vi "cv_03-03.vi"() -> ()   [LabVIEW 2013]
panel:
  out "SR - 3":dbl
  out "SR - 2":dbl
  out "SR - 1":dbl
  out "Feedback Before":dbl
  out "Feedback After":dbl
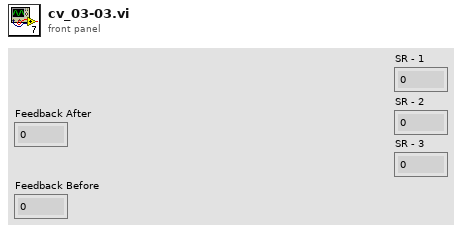
[diagram p1: front panel]
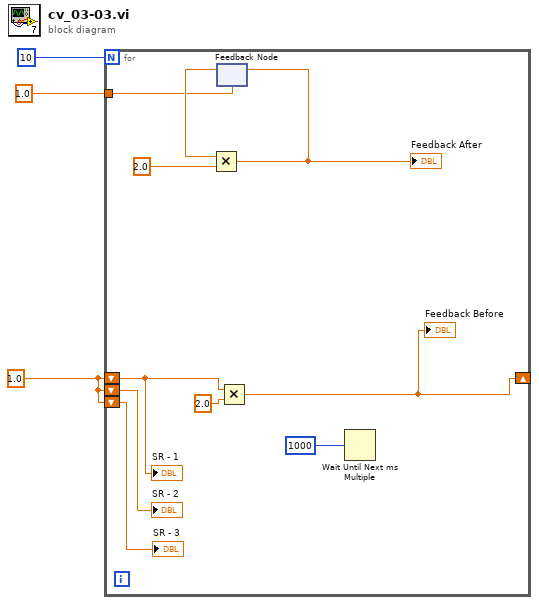
[diagram p0: block diagram]
diagram:
  w1 = 1.0
  n1 = for {
    N: 10 -> [_]
    tunnel: 1.0 -> [w8]
    shift-right: [w7] -> _
    shift-left: w1 -> [w6]
    shift-left: w1 -> [w5]
    shift-left: w1 -> [w4]
    n2 = feedback #1(w8) -> (w13:dbl)
    n3 = Multiply(x=w13, y=2.0) -> (x*y=w11:dbl)
    "Feedback After" <- w11
    n4 = feedback-in #1(w11) -> ()
    n5 = Multiply(x=w6, y=2.0) -> (x*y=w7:dbl)
    "Feedback Before" <- w7
    n6 = Wait Until Next ms Multiple(millisecond multiple=1000) -> ()  [unwired: 1 out]
    "SR - 1" <- w6
    "SR - 2" <- w5
    "SR - 3" <- w4
  }
